vi "Semaphore.vi"() -> ()   [LabVIEW 2011]
panel:
  in  "stop":bool
  out "当前任务":string
  out "Task 2#":dbl(graph)
  out "Task 1#":dbl(graph)
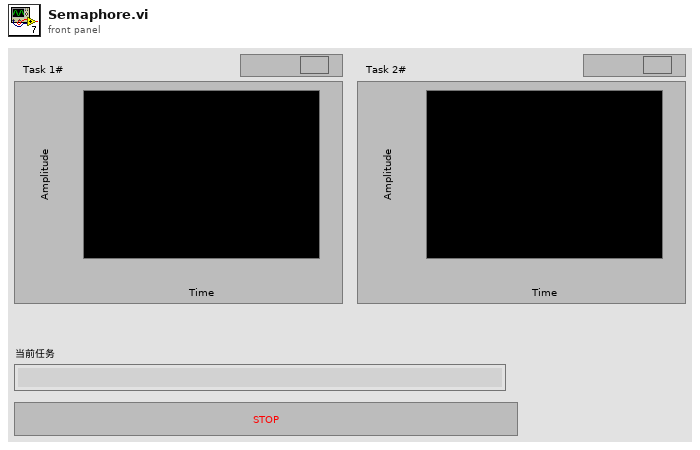
[diagram p1: front panel]
types:
  T1 = typedef "Semaphore RefNum" = refnum<k1>
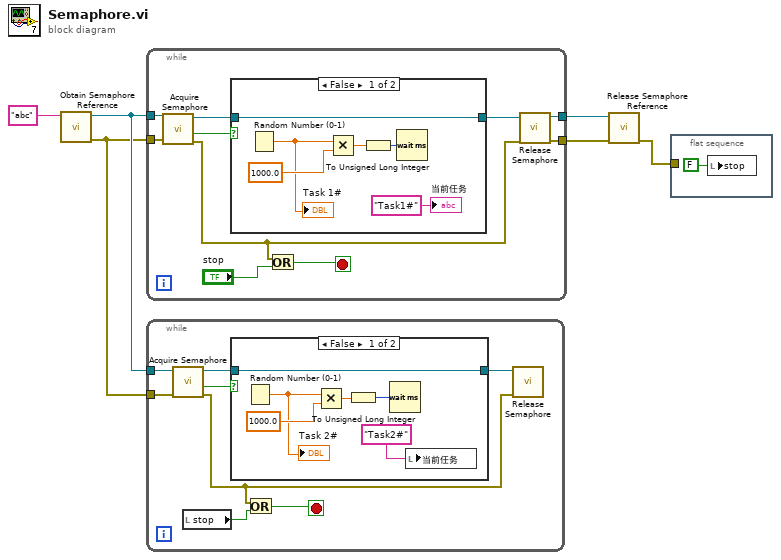
[diagram p0: block diagram]
diagram:
  n1 = call <vilib>:"Obtain Semaphore Reference.vi"("name (unnamed)"="abc") -> ("error out"=w4:errorcluster, "semaphore"=w5:T1)  [unwired: 4 in, 1 out]
  n2 = while {
    tunnel: w5 -> [w15]
    tunnel: w4 -> [w14]
    tunnel: [w8] -> w3
    tunnel: [w7] -> w2
    stop <- w9 stop-if-true
    n3 = call <vilib>:"Acquire Semaphore.vi"("error in (no error)"=w14, "semaphore"=w15) -> ("error out"=w11:errorcluster, "timed out"=w16:bool, "semaphore out"=w13:T1)  [unwired: 3 in]
    n4 = case shown="False" w16 {
      tunnel: [w22 w23] -> w12
      tunnel: w13 -> [w22 w23]
      frame False {
        n5 = Random Number (0-1)() -> (number: 0 to 1=w18:dbl)
        "Task 1#" <- w18
        n6 = Multiply(x=w18, y=1000.0) -> (x*y=w20:dbl)
        n7 = To Unsigned Long Integer(number=w20) -> (unsigned 32bit integer=w19:u32)
        n8 = Wait (ms)(milliseconds to wait=w19) -> ()  [unwired: 1 out]
        "当前任务" <- "Task1#" ("当前任务")
      }
      frame True {
      }
    }
    n9 = Or(x=w11, y="stop") -> (x .or. y?=w9:bool)
    n10 = call <vilib>:"Release Semaphore.vi"("error in (no error)"=w11, "semaphore"=w12) -> ("error out"=w7:errorcluster, "semaphore out"=w8:T1)  [unwired: 4 in]
  }
  n11 = while {
    tunnel: w5 -> [w30]
    tunnel: w4 -> [w29]
    stop <- w24 stop-if-true
    n12 = call <vilib>:"Acquire Semaphore.vi"("error in (no error)"=w29, "semaphore"=w30) -> ("error out"=w26:errorcluster, "timed out"=w31:bool, "semaphore out"=w28:T1)  [unwired: 3 in]
    n13 = local read "stop"() -> (w25:bool)
    n14 = case shown="False" w31 {
      tunnel: [w37 w38] -> w27
      tunnel: w28 -> [w37 w38]
      frame False {
        n15 = Random Number (0-1)() -> (number: 0 to 1=w34:dbl)
        "Task 2#" <- w34
        n16 = Multiply(x=w34, y=1000.0) -> (x*y=w36:dbl)
        n17 = To Unsigned Long Integer(number=w36) -> (unsigned 32bit integer=w33:u32)
        n18 = Wait (ms)(milliseconds to wait=w33) -> ()  [unwired: 1 out]
        n19 = local write "当前任务"("Task2#" ("当前任务")) -> ()
      }
      frame True {
      }
    }
    n20 = Or(x=w26, y=w25) -> (x .or. y?=w24:bool)
    n21 = call <vilib>:"Release Semaphore.vi"("error in (no error)"=w26, "semaphore"=w27) -> ()  [unwired: 4 in, 2 out]
  }
  n22 = call <vilib>:"Release Semaphore Reference.vi"("error in (no error)"=w2, "semaphore"=w3) -> ("error out"=w1:errorcluster)  [unwired: 8 in, 1 out]
  n23 = flat-sequence {
    tunnel: w1 -> [_]
    frame #0 {
      n24 = local write "stop"(FALSE ("stop")) -> ()
    }
  }
